vi "Find K24xx.vi"() -> ()   [LabVIEW 2014]
panel:
  in  "VISA 2":refnum<visa-resource-name>
  in  "VISA 1":refnum<visa-resource-name>
  in  "Serial Configuration":T1={"Baud Rate"=9600, "Parity"=0, "Data Bits"=8, "Stop Bits"=10, "Flow Control"=0} {"Flow Control" items=["None", "XON/XOFF", "RTS/CTS", "XON/XOFF & RTS/CTS", "DTR/DSR", "XON/XOFF & DTR/DSR"]; "Stop Bits" items=["1.0"=10, "1.5"=15, "2.0"=20]; "Data Bits" items=["7"=7, "8"=8]; "Parity" items=["None", "Odd", "Even", "Mark", "Space"]; "Baud Rate" items=["300"=300, "600"=600, "1200"=1200, "2400"=2400, "4800"=4800, "9600"=9600, "19200"=19200]}
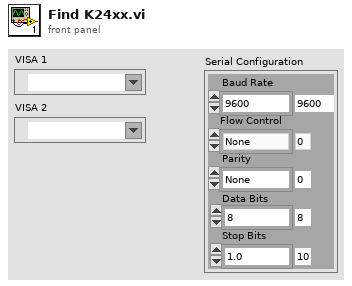
[diagram p1: front panel]
types:
  T1 = cluster{"Baud Rate":u32, "Parity":u16, "Data Bits":u16, "Stop Bits":u16, "Flow Control":u16}
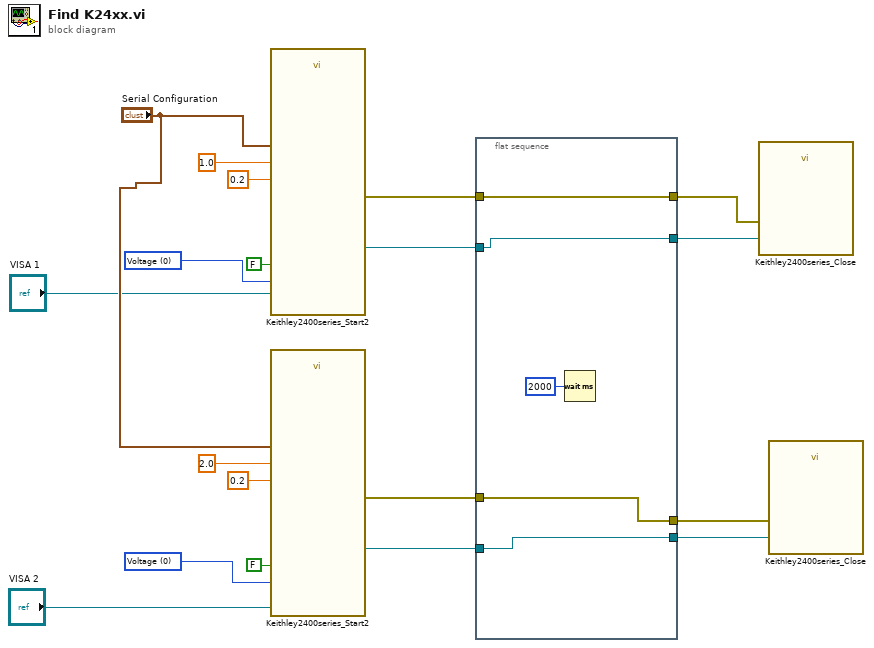
[diagram p0: block diagram]
diagram:
  w12 = u16 0 items=["Voltage", "Current"] ("Source Mode  (0: Voltage) in")
  w13 = u16 0 items=["Voltage", "Current"] ("Source Mode  (0: Voltage) in")
  n1 = call "Keithley2400series_Start2.vi"("Serial Configuration"="Serial Configuration", "Source Mode  (0: Voltage) in"=w13, "4W on"=FALSE, "Ограничение"=0.2, "Выход"=1.0, "VISA Refnum in"="VISA 1") -> ("error out"=w7:errorcluster, "VISA Refnum out"=w6:refnum<visa-resource-name>)  [unwired: 2 in, 2 out]
  n2 = call "Keithley2400series_Start2.vi"("Serial Configuration"="Serial Configuration", "Source Mode  (0: Voltage) in"=w12, "4W on"=FALSE, "Ограничение"=0.2, "Выход"=2.0, "VISA Refnum in"="VISA 2") -> ("error out"=w3:errorcluster, "VISA Refnum out"=w1:refnum<visa-resource-name>)  [unwired: 2 in, 2 out]
  n3 = flat-sequence {
    tunnel: [w23] -> w8
    tunnel: w7 -> [w23]
    tunnel: w6 -> [w22]
    tunnel: [w22] -> w5
    tunnel: [w21] -> w4
    tunnel: w3 -> [w21]
    tunnel: [w20] -> w2
    tunnel: w1 -> [w20]
    frame #0 {
      n4 = Wait (ms)(milliseconds to wait=u32 2000) -> ()  [unwired: 1 out]
    }
  }
  n5 = call "Keithley2400series_Close.vi"("error in (no error)"=w8, "VISA resource name"=w5) -> ()
  n6 = call "Keithley2400series_Close.vi"("error in (no error)"=w4, "VISA resource name"=w2) -> ()
